vi "Spectrum_Averaging.vi"(8 "error in":errorcluster, 9 "taille de la dimension":i32, 10 "Averages":u8=1 min=1, 11 "VISA resource name in":refnum<visa-resource-name>) -> (0 "error out":errorcluster, 1 "Saturated?":bool, 2 "XY Graph":cluster{dbl[], dbl[]}(graph), 3 "VISA resource name out":refnum<visa-resource-name>)   [LabVIEW 2023]
doc: "This VI acquires multiple spectra and provides the average as output"
uses:
  <instrlib>/Ocean Optics 2000 4000/Ocean Optics 2000 4000.lvlib
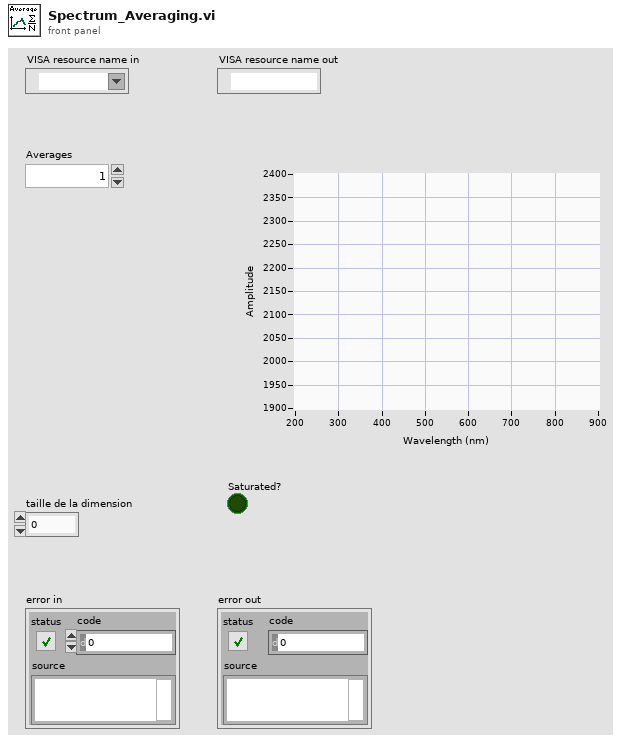
[diagram p1: front panel]
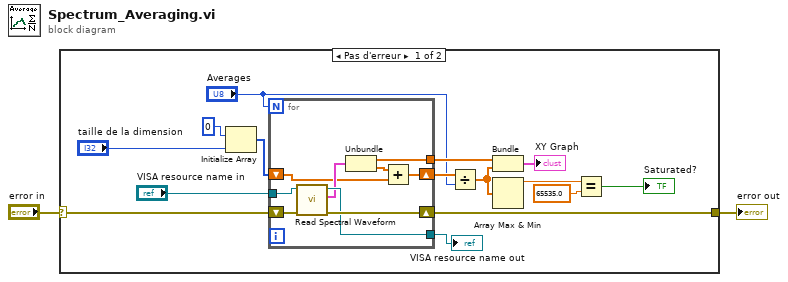
[diagram p0: block diagram]
diagram:
  n1 = case shown="Pas d'erreur" "error in" {
    selector: "error in" -> [w14 w27]
    tunnel: [w15 w27] -> w2
    frame No Error {
      n2 = Initialize Array(u16 0, "taille de la dimension") -> (w6:u16[])
      n3 = for {
        N: "Averages" -> [_]
        tunnel: [w25] -> w12
        tunnel: "VISA resource name in" -> [w24]
        shift-right: [w26] -> w15
        shift-left: w14 -> [w23]
        shift-right: [w20] -> w16
        shift-left: w6 -> [w19]
        tunnel: [w18] -> w17
        n4 = call <instrlib>:"Read Spectral Waveform.vi"("error in (no error)"=w23, "VISA resource name"=w24) -> ("error out"=w26:errorcluster, "Spectral Waveform"=w22:cluster{dbl[], dbl[]}, "VISA resource name out"=w25:refnum<visa-resource-name>)  [unwired: 7 in]
        n5 = Unbundle(w22) -> (w18:dbl[], w21:dbl[])
        n6 = Add(x=w21, y=w19) -> (x+y=w20:dbl[])
      }
      "VISA resource name out" <- w12
      n7 = Divide(x=w16, y="Averages") -> (x/y=w13:dbl[])
      n8 = Bundle(w17, w13) -> (→"XY Graph":cluster{dbl[], dbl[]})  [unwired: 1 in]
      n9 = Array Max & Min(array=w13) -> (max value=w4:dbl)  [unwired: 3 out]
      n10 = Equal?(x=w4, y=65535.0) -> (x = y?=→"Saturated?":bool)
    }
    frame Error {
    }
  }
  "error out" <- w2
